vi "PM2936R_DisplayDeviceInfo.vi"(3 "error in":errorcluster, 4 "DevInfoList In":refnum<k24>, 5 "Output Refnum In":refnum<vi>) -> (0 "error out":errorcluster, 1 "DevInfoList Out":refnum<k24>, 2 "Output Refnum Out":refnum<vi>)   [LabVIEW 2017]
uses:
  C:/Program Files (x86)/Newport/Newport USB Driver/Bin/UsbDllWrap.dll
  Program Files (x86)/Newport/Newport USB Driver/Bin/UsbDllWrap.dll
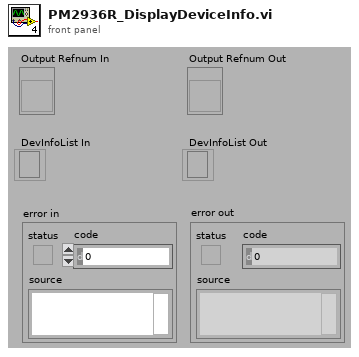
[diagram p1: front panel]
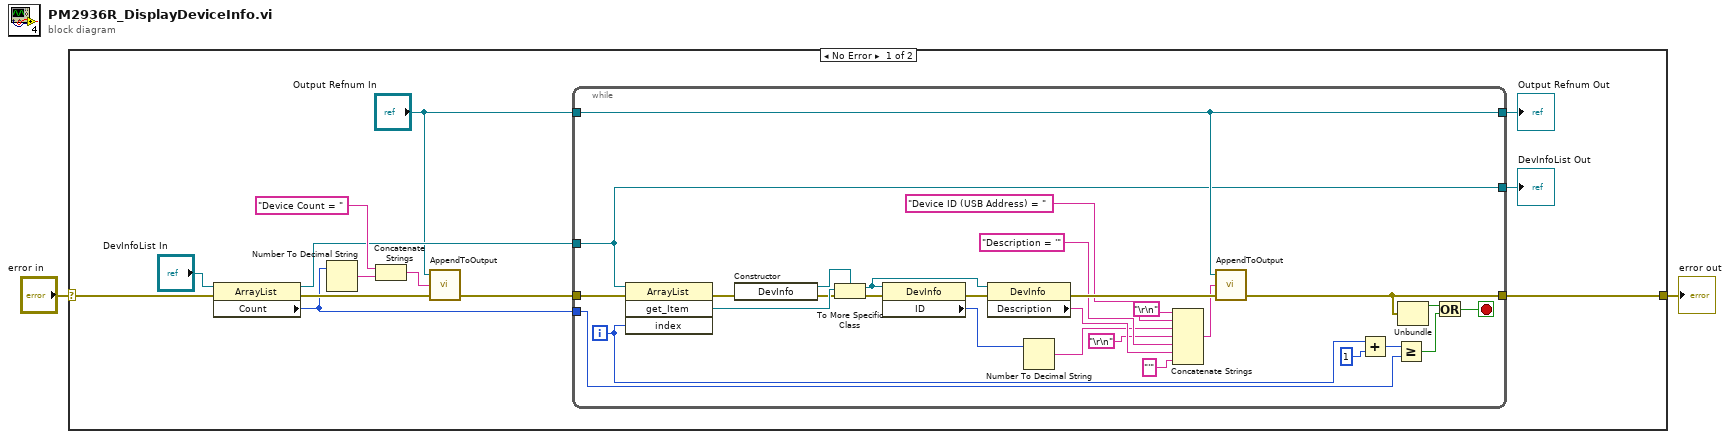
[diagram p0: block diagram]
diagram:
  n1 = case shown="No Error" "error in" {
    selector: "error in" -> [w3 w44]
    tunnel: [w7 w44] -> w2
    frame No Error {
      n2 = property class="ArrayList"(reference="DevInfoList In", error in=w3) -> (reference out=w10:refnum<k24>, error out=w11:errorcluster, "Count"=w8:i32)
      n3 = Number To Decimal String(number=w8) -> (decimal integer string=w15:string)  [unwired: 1 in]
      n4 = Concatenate Strings("Device Count = ", w15) -> (w13:string)
      n5 = call "AppendToOutput.vi"("error in"=w11, "Input String"=w13, "Output Refnum In"="Output Refnum In") -> ("error out"=w9:errorcluster)  [unwired: 1 in, 1 out]
      n6 = while {
        tunnel: "Output Refnum In" -> [w20]
        tunnel: w10 -> [w19]
        tunnel: w9 -> [w26]
        tunnel: w8 -> [w25]
        tunnel: [w21] -> w7
        tunnel: [w20] -> w6
        tunnel: [w19] -> w5
        i -> [w16]
        stop <- w24 stop-if-true
        n7 = invoke class="ArrayList" method="get_Item"(reference=w19, error in=w26, "index"=w16) -> (error out=w28:errorcluster, "get_Item"=w30:refnum<k24>)  [unwired: 1 in, 2 out]
        n8 = constructor class="DevInfo"(error in=w28) -> (reference out=w29:refnum<k24>, error out=w27:errorcluster)  [unwired: 2 in, 1 out]
        n9 = To More Specific Class(target class=w29, reference=w30, error in=w27) -> (specific class reference=w31:refnum<k24>, error out=w41:errorcluster)
        n10 = property class="DevInfo"(reference=w31, error in=w41) -> (error out=w42:errorcluster, "ID"=w32:i32)  [unwired: 1 out]
        n11 = property class="DevInfo"(reference=w31, error in=w42) -> (error out=w43:errorcluster, "Description"=w39:string)  [unwired: 1 out]
        n12 = Number To Decimal String(number=w32) -> (decimal integer string=w35:string)  [unwired: 1 in]
        n13 = Concatenate Strings("\r\n", "Device ID (USB Address) = ", w35, "\r\n", "Description = '", w39, "'") -> (w40:string)
        n14 = call "AppendToOutput.vi"("error in"=w43, "Input String"=w40, "Output Refnum In"=w20) -> ("error out"=w21:errorcluster)  [unwired: 1 in, 1 out]
        n15 = Add(x=w16, y=1) -> (x+y=w18:i32)
        n16 = Greater Or Equal?(x=w18, y=w25) -> (x >= y?=w22:bool)
        n17 = Unbundle(w21) -> ("status"=w23:bool)  [unwired: 2 out]
        n18 = Or(x=w23, y=w22) -> (x .or. y?=w24:bool)
      }
      "Output Refnum Out" <- w6
      "DevInfoList Out" <- w5
    }
    frame Error {
    }
  }
  "error out" <- w2
